vi "HLT.vi"(0 "System no.":i32=1 min=1 max=4 step=1, 2 "Affected axes":string[](array[string]), 3 "All axes?":bool, 4 "Axis identifier?":bool=TRUE, 5 "error in":errorcluster) -> (19 "error out":errorcluster)   [LabVIEW 2020]
doc: "GCS 3.0\n=====\n\nHLT (Halt Motion Smoothly)\n\nDescription\nActivates/deactivates the axis by switching its drive on/off.\nMotion of the axis is only possible if the axis is activated with EAX. Activating with EAX \npasses the axis from the Ready to switch state to the Operation enabled state. For further \ndetails, see \"Drive State Machine\". \n\nFormat\nHLT[{ <AxisID>}]\n\nArguments\nHLT without arguments stops all axes.\n<AxisID>\nAn axis of the controller\nPossible values: Alias of the axis\n\nResponse\nnone \n\nNotes\nHLT ends the following internal processes:\n- Reference move\nHLT can specifically stop one or more selected axes. In contrast to HLT, the STP command\nabruptly stops the motion and always applies to all axes.\nHLT does not cause a state transition in the drive state machine; for further details, see \"Drive \nState Machine\". \nIf multiple axes are addressed in the same HLT command and some of these axes are not in the \nOperation enabled state, HLT is executed for all axes in the Operation enabled state.\n\nUser command level\nUSR\n\n\nGCS 2.0\n=====\n\nStops motion of specified axes. HLT sets error code 10, call ERR?.vi to reset error after HLT has been called.\n\nC-413: If All axes? = TRUE, then Axis identifier? can be FALSE\nC-702: If All axes = TRUE, then Axis identifier must be TRUE\nC-843: If All axes = TRUE, then Axis identifier must be TRUE\nC-843.PM: If All axes = TRUE, then Axis identifier must be TRUE\nC-844: If All axes = TRUE, then Axis identifier must be TRUE\nC-848: If All axes = TRUE, then Axis identifier must be TRUE\nC-865: If All axes = TRUE, then Axis identifier can be FALSE\nC-866: If All axes? = TRUE, then Axis identifier? can be FALSE\nC-867: If All axes? = TRUE, then Axis identifier? can be FALSE\nC-877: If All axes? = TRUE, then Axis identifier? can be FALSE\nC-880: If All axes = TRUE, then Axis identifier must be TRUE\nC-884: If All axes? = TRUE, then Axis identifier? can be FALSE\nC-885: If All axes? = TRUE, then Axis identifier? can be FALSE\nC-886: If All axes? = TRUE, then Axis identifier? can be FALSE\nC-891: If All axes? = TRUE, then Axis identifier? must be TRUE\nE-517: If All axes? = TRUE, then Axis identifier? can be FALSE\nE-518: If All axes? = TRUE, then Axis identifier? can be FALSE\nE-710: If All axes? = TRUE, then Axis identifier? must be TRUE\nE-727: If All axes? = TRUE, then Axis identifier? must be TRUE\nE-754: If All axes? = TRUE, then Axis identifier? can be FALSE\nE-755: If All axes? = TRUE, then Axis identifier? must be TRUE\nE-761: If All axes = TRUE, then Axis identifier can be FALSE\nE-861: If All axes? = TRUE, then Axis identifier? can be FALSE\nE-871, E-872, E-873, E-874: If All axes? = TRUE, then Axis identifier? can be FALSE\nC-887, F-206, M-8X0: If All axes? = TRUE, then Axis identifier? can be FALSE. Only for GCS syntax version = GCS 2.0 or higher (check with CSV?.vi. If CSV?.vi is not supported, syntax version is GCS 1.0).\nHydra, Pollux: If All axes? = TRUE, then Axis identifier? can be FALSE. \nMercury: If All axes = TRUE, then Axis identifier can be FALSE\nMercury_GCS: If All axes? = TRUE, then Axis identifier? can be FALSE"
panel:
  # "HLT (Halt Motion Smoothly)\n\nActivates/deactivates the axis by switching its drive on/off.\nMotion of the axis is only possible if the axis is activated with EAX.\nActivating with EAX  passes the axis from the Ready to switch state\nto the Operation enabled state. For further details, see\n\"Drive State Machine\"."
  # "Halt"
  # "If all axes: use"
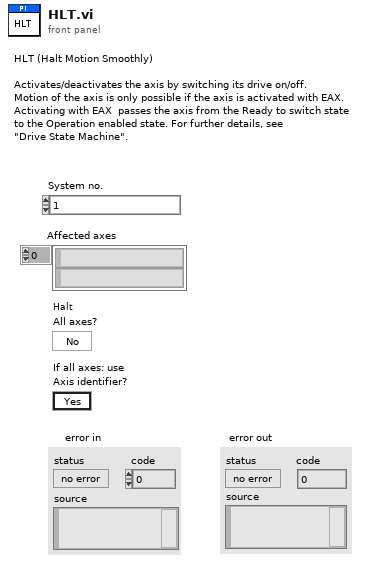
[diagram p1: front panel]
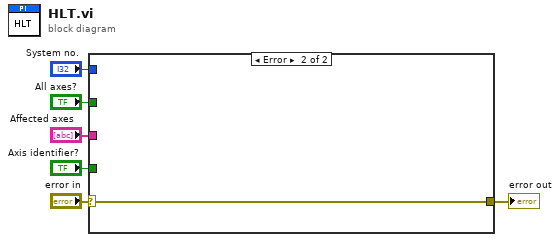
[diagram p0: block diagram]
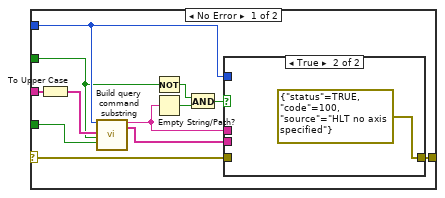
[diagram p2: hidden frame]
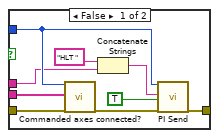
[diagram p3: hidden frame]
diagram:
  n1 = case shown="Error" "error in" {
    selector: "error in" -> [w11 w29]
    tunnel: "Affected axes" -> [w18 _]
    tunnel: [w12 w29] -> w5
    tunnel: "Axis identifier?" -> [w16 _]
    tunnel: "System no." -> [w15 _]
    tunnel: "All axes?" -> [w14 _]
    frame No Error {
      n2 = To Upper Case(1:w18) -> (0:w17:string[])
      n3 = call "Build query command substring.vi"("System no."=w15, "Axes to query in"=w17, "Query\nAll axes?"=w14, "For all axes: use\nAxis identifier?"=w16) -> ("Command substring"=w8:string, "Axes to query out"=w10:string[])  [unwired: 2 in, 12 out]
      n4 = Not(x=w14) -> (.not. x?=w13:bool)
      n5 = Empty String/Path?(string/path=w8) -> (empty?=w9:bool)
      n6 = And(x=w13, y=w9) -> (x .and. y?=w7:bool)
      n7 = case shown="True" w7 {
        tunnel: w15 -> [w24 _]
        tunnel: [w23 errorcluster {"status"=TRUE, "code"=100, "source"="HLT no axis specified"} ("error out")] -> w12
        tunnel: w11 -> [w22 _]
        tunnel: w10 -> [w21 _]
        tunnel: w8 -> [w19 _]
        frame False {
          n8 = call "Commanded axes connected?.vi"("System no."=w24, "Commanded axes"=w21, "error in"=w22) -> ("error out"=w20:errorcluster)  [unwired: 1 in, 15 out]
          n9 = Concatenate Strings("HLT ", w19) -> (w25:string)
          n10 = call "PI Send.vi"("System no."=w24, "String to send"=w25, "Attach termination char.?"=TRUE ("Attach Linefeed?"), "error in"=w20) -> ("error out"=w23:errorcluster)  [unwired: 2 in, 13 out]
        }
        frame True {
        }
      }
    }
    frame Error {
    }
  }
  "error out" <- w5
